vi "BCU诊断标定.vi"(8 "CAN端口":u16(ring), 9 "设备索引号":u16(ring), 10 "CAN卡类型":u32(ring)=21, 11 "Myindex":dbl=1.0) -> (3 "成功":bool)   [LabVIEW 2013] (continued)
                        n2401 = local write "风机继电器(从)"(w2943) -> ()
                        n2402 = One Button Dialog(message="继电器处理超时" ("消息"), button name ("OK")="是" ("按钮名称（“确定”）")) -> ()  [unwired: 1 out]
                      }
                      frame True {
                      }
                    }
                  }
                }
              }
            }
          }
          event "DO1": Value Change {
            n2403 = event-data() -> ("NewVal"=w2947:bool)  [unwired: 6 out]
            n2404 = stacked-sequence {
              tunnel: w2947 -> [_ w2960 _]
              frame #0 {
                w2950 = FALSE ("清BUFF")
                n2405 = local write "继电器超时处理"(FALSE ("继电器超时处理")) -> ()
                n2406 = local write "清BUFF"(w2950) -> ()
                n2407 = local write "正级继电器 9"(w2950) -> ()
                n2408 = local write "主从选择"(enum32{"主板", "从板"}."主板" ("主从选择")) -> ()
              }
              frame #1 {
                n2409 = case shown="真" w2960 {
                  selector: w2960 -> [w2975 w2995]
                  tunnel: [w2974 w2994] -> w2959
                  tunnel: [w2962 w2982] -> w2954
                  frame False {
                    w2970 = 256.0 ("y")
                    w2962 = u32 2 ("命令序号")
                    w2974 = u8 192 ("命令")
                    n2410 = local read "动作保持时间"() -> (w2971:dbl)
                    n2411 = Quotient & Remainder(x=w2971, y=w2970) -> (x-y*floor(x/y)=w2963:dbl, floor(x/y)=w2967:dbl)
                    n2412 = Quotient & Remainder(x=w2967, y=w2970) -> (x-y*floor(x/y)=w2964:dbl, floor(x/y)=w2968:dbl)
                    n2413 = Quotient & Remainder(x=w2968, y=w2970) -> (x-y*floor(x/y)=w2965:dbl, floor(x/y)=w2969:dbl)
                    n2414 = local read "设备索引号"() -> (w2979:u16)
                    n2415 = local read "CAN卡类型"() -> (w2980:u32)
                    n2416 = local read "CAN端口"() -> (w2978:u16)
                    n2417 = Boolean To (0,1)(Boolean=w2975) -> (0, 1=w2972:i16)
                    n2418 = Quotient & Remainder(x=w2969, y=w2970) -> (x-y*floor(x/y)=w2966:dbl)  [unwired: 1 out]
                    n2419 = Build Array(i16 1 ("元素"), w2972, w2966, w2965, w2964, w2963, 0.0 ("元素")) -> (w2976:dbl[])
                    n2420 = call "多帧发送机制(EV05).vi"("can卡类型"=w2980, "设备索引号"=w2979, "CAN端口"=w2978, "命令"=w2974, "板号"=u8 0, "命令序号"=w2962, "输入数据"=w2976) -> ()  [unwired: 2 in, 11 out]
                  }
                  frame True {
                    w2990 = 256.0 ("y")
                    w2982 = u32 2 ("命令序号")
                    w2994 = u8 192 ("命令")
                    n2421 = local read "动作保持时间"() -> (w2991:dbl)
                    n2422 = Quotient & Remainder(x=w2991, y=w2990) -> (x-y*floor(x/y)=w2983:dbl, floor(x/y)=w2987:dbl)
                    n2423 = Quotient & Remainder(x=w2987, y=w2990) -> (x-y*floor(x/y)=w2984:dbl, floor(x/y)=w2988:dbl)
                    n2424 = Quotient & Remainder(x=w2988, y=w2990) -> (x-y*floor(x/y)=w2985:dbl, floor(x/y)=w2989:dbl)
                    n2425 = local read "设备索引号"() -> (w2999:u16)
                    n2426 = local read "CAN卡类型"() -> (w3000:u32)
                    n2427 = local read "CAN端口"() -> (w2998:u16)
                    n2428 = Boolean To (0,1)(Boolean=w2995) -> (0, 1=w2992:i16)
                    n2429 = Quotient & Remainder(x=w2989, y=w2990) -> (x-y*floor(x/y)=w2986:dbl)  [unwired: 1 out]
                    n2430 = Build Array(i16 1 ("元素"), w2992, w2986, w2985, w2984, w2983, 0.0 ("元素")) -> (w2996:dbl[])
                    n2431 = call "多帧发送机制(EV05).vi"("can卡类型"=w3000, "设备索引号"=w2999, "CAN端口"=w2998, "命令"=w2994, "板号"=u8 0, "命令序号"=w2982, "输入数据"=w2996) -> ()  [unwired: 2 in, 11 out]
                  }
                }
                n2432 = local write "命令序号"(w2954) -> ()
                n2433 = local write "命令"(w2959) -> ()
                n2434 = local write "控制1"(TRUE ("控制1")) -> ()
                n2435 = local write "写?"(FALSE ("写?")) -> ()
                n2436 = local write "消除"(TRUE ("消除")) -> ()
                n2437 = global write "EV05全局变量1.vi" "流控帧 2"(TRUE ("流控帧 2")) -> ()
                n2438 = global write "EV05全局变量1.vi" "流控帧"(FALSE ("流控帧")) -> ()
              }
              frame #2 {
                n2439 = flat-sequence {
                  tunnel: [w3002] -> w3001
                  tunnel: w3001 -> [w3009]
                  frame #0 {
                    n2440 = while {
                      tunnel: [w3003] -> w3002
                      i -> [w3007]
                      stop <- w3004 stop-if-true
                      n2441 = local read "继电器超时处理"() -> (w3003:bool)
                      n2442 = Greater Or Equal?(x=w3007, y=20) -> (x >= y?=w3005:bool)
                      n2443 = Wait Until Next ms Multiple(millisecond multiple=u32 100 ("毫秒倍数")) -> ()  [unwired: 1 out]
                      n2444 = Or(x=w3003, y=w3005) -> (x .or. y?=w3004:bool)
                    }
                  }
                  frame #1 {
                    n2445 = case shown="假" w3009 {
                      frame False {
                        n2446 = local read "DO1"() -> (w3011:bool)
                        n2447 = Not(x=w3011) -> (.not. x?=w3010:bool)
                        n2448 = local write "DO1"(w3010) -> ()
                        n2449 = One Button Dialog(message="DO控制处理超时" ("消息"), button name ("OK")="是" ("按钮名称（“确定”）")) -> ()  [unwired: 1 out]
                      }
                      frame True {
                      }
                    }
                  }
                }
              }
            }
          }
          event "DO2": Value Change {
            n2450 = event-data() -> ("NewVal"=w3014:bool)  [unwired: 6 out]
            n2451 = stacked-sequence {
              tunnel: w3014 -> [_ w3027 _]
              frame #0 {
                w3017 = FALSE ("清BUFF")
                n2452 = local write "继电器超时处理"(FALSE ("继电器超时处理")) -> ()
                n2453 = local write "主从选择"(enum32{"主板", "从板"}."主板" ("主从选择")) -> ()
                n2454 = local write "清BUFF"(w3017) -> ()
                n2455 = local write "正级继电器 10"(w3017) -> ()
              }
              frame #1 {
                n2456 = case shown="真" w3027 {
                  selector: w3027 -> [w3042 w3062]
                  tunnel: [w3041 w3061] -> w3026
                  tunnel: [w3029 w3049] -> w3021
                  frame False {
                    w3037 = 256.0 ("y")
                    w3029 = u32 2 ("命令序号")
                    w3041 = u8 192 ("命令")
                    n2457 = local read "动作保持时间"() -> (w3038:dbl)
                    n2458 = Quotient & Remainder(x=w3038, y=w3037) -> (x-y*floor(x/y)=w3030:dbl, floor(x/y)=w3034:dbl)
                    n2459 = Quotient & Remainder(x=w3034, y=w3037) -> (x-y*floor(x/y)=w3031:dbl, floor(x/y)=w3035:dbl)
                    n2460 = Quotient & Remainder(x=w3035, y=w3037) -> (x-y*floor(x/y)=w3032:dbl, floor(x/y)=w3036:dbl)
                    n2461 = local read "设备索引号"() -> (w3046:u16)
                    n2462 = local read "CAN卡类型"() -> (w3047:u32)
                    n2463 = local read "CAN端口"() -> (w3045:u16)
                    n2464 = Boolean To (0,1)(Boolean=w3042) -> (0, 1=w3039:i16)
                    n2465 = Quotient & Remainder(x=w3036, y=w3037) -> (x-y*floor(x/y)=w3033:dbl)  [unwired: 1 out]
                    n2466 = Build Array(i16 2 ("元素"), w3039, w3033, w3032, w3031, w3030, 0.0 ("元素")) -> (w3043:dbl[])
                    n2467 = call "多帧发送机制(EV05).vi"("can卡类型"=w3047, "设备索引号"=w3046, "CAN端口"=w3045, "命令"=w3041, "板号"=u8 0, "命令序号"=w3029, "输入数据"=w3043) -> ()  [unwired: 2 in, 11 out]
                  }
                  frame True {
                    w3057 = 256.0 ("y")
                    w3049 = u32 2 ("命令序号")
                    w3061 = u8 192 ("命令")
                    n2468 = local read "动作保持时间"() -> (w3058:dbl)
                    n2469 = Quotient & Remainder(x=w3058, y=w3057) -> (x-y*floor(x/y)=w3050:dbl, floor(x/y)=w3054:dbl)
                    n2470 = Quotient & Remainder(x=w3054, y=w3057) -> (x-y*floor(x/y)=w3051:dbl, floor(x/y)=w3055:dbl)
                    n2471 = Quotient & Remainder(x=w3055, y=w3057) -> (x-y*floor(x/y)=w3052:dbl, floor(x/y)=w3056:dbl)
                    n2472 = local read "设备索引号"() -> (w3066:u16)
                    n2473 = local read "CAN卡类型"() -> (w3067:u32)
                    n2474 = local read "CAN端口"() -> (w3065:u16)
                    n2475 = Boolean To (0,1)(Boolean=w3062) -> (0, 1=w3059:i16)
                    n2476 = Quotient & Remainder(x=w3056, y=w3057) -> (x-y*floor(x/y)=w3053:dbl)  [unwired: 1 out]
                    n2477 = Build Array(i16 2 ("元素"), w3059, w3053, w3052, w3051, w3050, 0.0 ("元素")) -> (w3063:dbl[])
                    n2478 = call "多帧发送机制(EV05).vi"("can卡类型"=w3067, "设备索引号"=w3066, "CAN端口"=w3065, "命令"=w3061, "板号"=u8 0, "命令序号"=w3049, "输入数据"=w3063) -> ()  [unwired: 2 in, 11 out]
                  }
                }
                n2479 = local write "命令序号"(w3021) -> ()
                n2480 = local write "命令"(w3026) -> ()
                n2481 = local write "控制1"(TRUE ("控制1")) -> ()
                n2482 = local write "写?"(FALSE ("写?")) -> ()
                n2483 = local write "消除"(TRUE ("消除")) -> ()
                n2484 = global write "EV05全局变量1.vi" "流控帧 2"(TRUE ("流控帧 2")) -> ()
                n2485 = global write "EV05全局变量1.vi" "流控帧"(FALSE ("流控帧")) -> ()
              }
              frame #2 {
                n2486 = flat-sequence {
                  tunnel: [w3069] -> w3068
                  tunnel: w3068 -> [w3076]
                  frame #0 {
                    n2487 = while {
                      tunnel: [w3070] -> w3069
                      i -> [w3074]
                      stop <- w3071 stop-if-true
                      n2488 = local read "继电器超时处理"() -> (w3070:bool)
                      n2489 = Greater Or Equal?(x=w3074, y=20) -> (x >= y?=w3072:bool)
                      n2490 = Wait Until Next ms Multiple(millisecond multiple=u32 100 ("毫秒倍数")) -> ()  [unwired: 1 out]
                      n2491 = Or(x=w3070, y=w3072) -> (x .or. y?=w3071:bool)
                    }
                  }
                  frame #1 {
                    n2492 = case shown="假" w3076 {
                      frame False {
                        n2493 = local read "DO2"() -> (w3078:bool)
                        n2494 = Not(x=w3078) -> (.not. x?=w3077:bool)
                        n2495 = local write "DO2"(w3077) -> ()
                        n2496 = One Button Dialog(message="DO控制处理超时" ("消息"), button name ("OK")="是" ("按钮名称（“确定”）")) -> ()  [unwired: 1 out]
                      }
                      frame True {
                      }
                    }
                  }
                }
              }
            }
          }
          event "DO1 2": Value Change {
            n2497 = event-data() -> ("NewVal"=w3081:bool)  [unwired: 6 out]
            n2498 = stacked-sequence {
              tunnel: w3081 -> [_ w3095 _]
              frame #0 {
                w3084 = FALSE ("继电器超时处理")
                n2499 = local write "继电器超时处理"(w3084) -> ()
                n2500 = local write "正级继电器 11"(w3084) -> ()
                n2501 = local write "主从选择"(enum32{"主板", "从板"}."从板" ("主从选择")) -> ()
              }
              frame #1 {
                n2502 = case shown="假" w3095 {
                  selector: w3095 -> [w3110 w3130]
                  tunnel: [w3109 w3129] -> w3094
                  tunnel: [w3108 w3128] -> w3088
                  tunnel: [w3097 w3117] -> w3089
                  frame True {
                    w3105 = 256.0 ("y")
                    w3097 = u32 2 ("命令序号")
                    w3109 = u8 192 ("命令")
                    n2503 = local read "动作保持时间"() -> (w3106:dbl)
                    n2504 = Quotient & Remainder(x=w3106, y=w3105) -> (x-y*floor(x/y)=w3098:dbl, floor(x/y)=w3102:dbl)
                    n2505 = Quotient & Remainder(x=w3102, y=w3105) -> (x-y*floor(x/y)=w3099:dbl, floor(x/y)=w3103:dbl)
                    n2506 = Quotient & Remainder(x=w3103, y=w3105) -> (x-y*floor(x/y)=w3100:dbl, floor(x/y)=w3104:dbl)
                    n2507 = Quotient & Remainder(x=w3104, y=w3105) -> (x-y*floor(x/y)=w3101:dbl)  [unwired: 1 out]
                    n2508 = Boolean To (0,1)(Boolean=w3110) -> (0, 1=w3107:i16)
                    n2509 = local read "设备索引号"() -> (w3114:u16)
                    n2510 = local read "CAN卡类型"() -> (w3115:u32)
                    n2511 = local read "从板板号"() -> (w3108:u8)
                    n2512 = local read "CAN端口"() -> (w3113:u16)
                    n2513 = Build Array(i16 3 ("元素"), w3107, w3101, w3100, w3099, w3098, 0.0 ("元素")) -> (w3112:dbl[])
                    n2514 = call "多帧发送机制(EV05).vi"("can卡类型"=w3115, "设备索引号"=w3114, "CAN端口"=w3113, "命令"=w3109, "板号"=w3108, "命令序号"=w3097, "输入数据"=w3112) -> ()  [unwired: 2 in, 11 out]
                  }
                  frame False {
                    w3125 = 256.0 ("y")
                    w3117 = u32 2 ("命令序号")
                    w3129 = u8 192 ("命令")
                    n2515 = local read "动作保持时间"() -> (w3126:dbl)
                    n2516 = Quotient & Remainder(x=w3126, y=w3125) -> (x-y*floor(x/y)=w3118:dbl, floor(x/y)=w3122:dbl)
                    n2517 = Quotient & Remainder(x=w3122, y=w3125) -> (x-y*floor(x/y)=w3119:dbl, floor(x/y)=w3123:dbl)
                    n2518 = Quotient & Remainder(x=w3123, y=w3125) -> (x-y*floor(x/y)=w3120:dbl, floor(x/y)=w3124:dbl)
                    n2519 = Quotient & Remainder(x=w3124, y=w3125) -> (x-y*floor(x/y)=w3121:dbl)  [unwired: 1 out]
                    n2520 = Boolean To (0,1)(Boolean=w3130) -> (0, 1=w3127:i16)
                    n2521 = local read "设备索引号"() -> (w3134:u16)
                    n2522 = local read "CAN卡类型"() -> (w3135:u32)
                    n2523 = local read "从板板号"() -> (w3128:u8)
                    n2524 = local read "CAN端口"() -> (w3133:u16)
                    n2525 = Build Array(i16 1 ("元素"), w3127, w3121, w3120, w3119, w3118, 0.0 ("元素")) -> (w3132:dbl[])
                    n2526 = call "多帧发送机制(EV05).vi"("can卡类型"=w3135, "设备索引号"=w3134, "CAN端口"=w3133, "命令"=w3129, "板号"=w3128, "命令序号"=w3117, "输入数据"=w3132) -> ()  [unwired: 2 in, 11 out]
                  }
                }
                n2527 = local write "从板板号"(w3088) -> ()
                n2528 = local write "命令序号"(w3089) -> ()
                n2529 = local write "命令"(w3094) -> ()
                n2530 = local write "清BUFF"(FALSE ("清BUFF")) -> ()
                n2531 = local write "写?"(FALSE ("写?")) -> ()
                n2532 = local write "控制1"(TRUE ("控制1")) -> ()
                n2533 = global write "EV05全局变量1.vi" "流控帧"(FALSE ("流控帧")) -> ()
                n2534 = global write "EV05全局变量1.vi" "流控帧 2"(TRUE ("流控帧 2")) -> ()
                n2535 = local write "消除"(TRUE ("消除")) -> ()
              }
              frame #2 {
                n2536 = flat-sequence {
                  tunnel: [w3137] -> w3136
                  tunnel: w3136 -> [w3144]
                  frame #0 {
                    n2537 = while {
                      tunnel: [w3138] -> w3137
                      i -> [w3142]
                      stop <- w3139 stop-if-true
                      n2538 = local read "继电器超时处理"() -> (w3138:bool)
                      n2539 = Greater Or Equal?(x=w3142, y=20) -> (x >= y?=w3140:bool)
                      n2540 = Wait Until Next ms Multiple(millisecond multiple=u32 100 ("毫秒倍数")) -> ()  [unwired: 1 out]
                      n2541 = Or(x=w3138, y=w3140) -> (x .or. y?=w3139:bool)
                    }
                  }
                  frame #1 {
                    n2542 = case shown="假" w3144 {
                      frame False {
                        n2543 = local read "DO1 2"() -> (w3146:bool)
                        n2544 = Not(x=w3146) -> (.not. x?=w3145:bool)
                        n2545 = local write "DO1 2"(w3145) -> ()
                        n2546 = One Button Dialog(message="DO控制处理超时" ("消息"), button name ("OK")="是" ("按钮名称（“确定”）")) -> ()  [unwired: 1 out]
                      }
                      frame True {
                      }
                    }
                  }
                }
              }
            }
          }
          event "读取转换为写入": Value Change {
            n2547 = event-data() -> ("NewVal"=w3149:bool)  [unwired: 6 out]
            n2548 = case shown="真" w3149 {
              tunnel: w3153 -> [w3155 w3160]
              tunnel: [w3155 w3159] -> w3152
              tunnel: w3151 -> [w3154 w3158]
              tunnel: [w3154 w3157] -> w3150
              frame False {
              }
              frame True {
                n2549 = Enqueue Element(queue=w3160, element="读取转换为写入", error in (no error)=w3158) -> (queue out=w3159:refnum<queue>, error out=w3157:errorcluster)  [unwired: 2 out]
              }
            }
          }
          event "读取故障详细状态": Value Change {
            n2550 = event-data() -> ("NewVal"=w3165:bool)  [unwired: 5 out]
            n2551 = case shown="真" w3165 {
              tunnel: w3164 -> [w3167 w3180]
              tunnel: w3163 -> [w3166 w3179]
              tunnel: [w3167 w3178] -> w3162
              tunnel: [w3166 w3177] -> w3161
              frame False {
              }
              frame True {
                n2552 = disable-structure shown="启用" {
                  disable-tunnel: [w3189 TRUE ("发送成功")] -> w3176
                  frame Disabled {
                    n2553 = local read "主从选择"() -> (w3181:enum32{"主板", "从板"})
                    n2554 = case shown="\"主板\", 默认" w3181 {
                      tunnel: [0.0 ("FUNC") w3191] -> w3186
                      frame "主板", Default {
                      }
                      frame "从板" {
                        n2555 = local read "从板号"() -> (w3191:u8)
                      }
                    }
                    n2556 = local read "设备索引号"() -> (w3183:u16)
                    n2557 = local read "CAN卡类型"() -> (w3184:u32)
                    n2558 = local read "CAN端口"() -> (w3182:u16)
                    n2559 = call "标定授权发送.vi"("CAN卡类型"=w3184, "解锁类型"=enum16{"读取", "写", "下载"}."写", "设备索引号"=w3183, "CAN端口"=w3182, "是否连接"=TRUE, "板选择"=0, "FUNC"=w3186) -> ("发送成功"=w3189:bool)  [unwired: 8 out]
                  }
                  frame Enabled {
                  }
                }
                n2560 = case shown="真" w3176 {
                  tunnel: w3180 -> [w3194 w3199]
                  tunnel: w3179 -> [w3193 w3198]
                  tunnel: [w3194 w3196] -> w3178
                  tunnel: [w3193 w3195] -> w3177
                  frame False {
                  }
                  frame True {
                    n2561 = Enqueue Element(queue=w3199, element="读取故障状态" ("元素"), error in (no error)=w3198) -> (queue out=w3196:refnum<queue>, error out=w3195:errorcluster)  [unwired: 2 out]
                  }
                }
                n2562 = local write "电池故障"(string[][] []) -> ()
                n2563 = global write "EV05全局变量1.vi" "流控帧 2"(TRUE ("流控帧")) -> ()
                n2564 = local write "写?"(FALSE ("写?")) -> ()
                n2565 = local write "控制1"(TRUE ("控制1")) -> ()
                n2566 = local write "消除"(TRUE ("消除")) -> ()
                n2567 = local write "清BUFF"(FALSE ("清BUFF")) -> ()
                n2568 = global write "EV05全局变量1.vi" "流控帧"(FALSE ("流控帧")) -> ()
                n2569 = call <vilib>:"Set Busy.vi"("disable click? (T)"=FALSE) -> ()  [unwired: 3 in, 8 out]
              }
            }
          }
          event "项目软本读取": Value Change {
            n2570 = event-data() -> ("NewVal"=w3204:bool)  [unwired: 5 out]
            n2571 = case shown="真" w3204 {
              tunnel: w3203 -> [w3206 w3213]
              tunnel: w3202 -> [w3205 w3212]
              tunnel: [w3206 w3211] -> w3201
              tunnel: [w3205 w3210] -> w3200
              frame False {
              }
              frame True {
                n2572 = global read "EV05全局变量1.vi" "授权功能"() -> (w3208:bool)
                n2573 = case shown="假" w3208 {
                  tunnel: [TRUE ("发送成功") w3232] -> w3209
                  frame False {
                  }
                  frame True {
                    n2574 = local read "设备索引号"() -> (w3227:u16)
                    n2575 = local read "CAN卡类型"() -> (w3228:u32)
                    n2576 = local read "CAN端口"() -> (w3226:u16)
                    n2577 = call "标定授权发送.vi"("CAN卡类型"=w3228, "解锁类型"=enum16{"读取", "写", "下载"}."读取", "设备索引号"=w3227, "CAN端口"=w3226, "是否连接"=TRUE, "板选择"=0, "FUNC"=u32 0) -> ("发送成功"=w3232:bool)  [unwired: 8 out]
                  }
                }
                n2578 = stacked-sequence {
                  tunnel: [w3216] -> w3207
                  frame #0 {
                    w3216 = FALSE ("disable click? (T)")
                    w3219 = FALSE ("写?")
                    n2579 = local write "写?"(w3219) -> ()
                    n2580 = global write "EV05全局变量1.vi" "写入超时"(w3219) -> ()
                    n2581 = local write "项目软件版本号"(" " ("项目软件版本号")) -> ()
                    n2582 = global write "EV05全局变量1.vi" "流控帧"(FALSE ("流控帧")) -> ()
                    n2583 = local write "主从选择"(enum32{"主板", "从板"}."主板" ("主从选择")) -> ()
                    n2584 = call <vilib>:"Set Busy.vi"("disable click? (T)"=w3216) -> ()  [unwired: 3 in, 8 out]
                    n2585 = local write "清BUFF"(FALSE ("清BUFF")) -> ()
                    n2586 = property on="保存版本信息" class="Bool (严格)"("Visible"=TRUE ("可见")) -> ()  [unwired: 2 in, 2 out]
                    n2587 = global write "EV05全局变量1.vi" "流控帧 2"(TRUE ("流控帧 2")) -> ()
                    n2588 = local write "控制1"(TRUE ("控制1")) -> ()
                    n2589 = local write "消除"(TRUE ("消除")) -> ()
                  }
                }
                n2590 = case shown="真" w3209 {
                  tunnel: w3213 -> [w3234 w3239]
                  tunnel: w3212 -> [w3233 w3238]
                  tunnel: [w3234 w3236] -> w3211
                  tunnel: [w3233 w3235] -> w3210
                  tunnel: w3207 -> [_ _]
                  frame False {
                  }
                  frame True {
                    n2591 = Enqueue Element(queue=w3239, element="项目软件版本读取" ("元素"), error in (no error)=w3238) -> (queue out=w3236:refnum<queue>, error out=w3235:errorcluster)  [unwired: 2 out]
                  }
                }
              }
            }
          }
          event "读硬件版本号": Value Change {
            n2592 = event-data() -> ("NewVal"=w3244:bool)  [unwired: 5 out]
            n2593 = case shown="真" w3244 {
              tunnel: w3243 -> [w3246 w3253]
              tunnel: w3242 -> [w3245 w3252]
              tunnel: [w3246 w3251] -> w3241
              tunnel: [w3245 w3250] -> w3240
              frame False {
              }
              frame True {
                n2594 = global read "EV05全局变量1.vi" "授权功能"() -> (w3248:bool)
                n2595 = case shown="假" w3248 {
                  tunnel: [TRUE ("发送成功") w3272] -> w3249
                  frame False {
                  }
                  frame True {
                    n2596 = local read "设备索引号"() -> (w3267:u16)
                    n2597 = local read "CAN卡类型"() -> (w3268:u32)
                    n2598 = local read "CAN端口"() -> (w3266:u16)
                    n2599 = call "标定授权发送.vi"("CAN卡类型"=w3268, "解锁类型"=enum16{"读取", "写", "下载"}."读取", "设备索引号"=w3267, "CAN端口"=w3266, "是否连接"=TRUE, "板选择"=0, "FUNC"=u32 0) -> ("发送成功"=w3272:bool)  [unwired: 8 out]
                  }
                }
                n2600 = stacked-sequence {
                  tunnel: [w3256] -> w3247
                  frame #0 {
                    w3256 = TRUE ("控制1")
                    w3260 = FALSE ("写?")
                    n2601 = local write "写?"(w3260) -> ()
                    n2602 = global write "EV05全局变量1.vi" "写入超时"(w3260) -> ()
                    n2603 = call <vilib>:"Set Busy.vi"("disable click? (T)"=FALSE) -> ()  [unwired: 3 in, 8 out]
                    n2604 = local write "硬件版本号"("" ("硬件版本号")) -> ()
                    n2605 = property on="保存版本信息" class="Bool (严格)"("Visible"=TRUE ("可见")) -> ()  [unwired: 2 in, 2 out]
                    n2606 = local write "主从选择"(enum32{"主板", "从板"}."主板" ("主从选择")) -> ()
                    n2607 = local write "控制1"(w3256) -> ()
                    n2608 = local write "清BUFF"(FALSE ("清BUFF")) -> ()
                    n2609 = global write "EV05全局变量1.vi" "流控帧 2"(TRUE ("流控帧 2")) -> ()
                    n2610 = local write "消除"(TRUE ("消除")) -> ()
                    n2611 = global write "EV05全局变量1.vi" "流控帧"(FALSE ("流控帧")) -> ()
                  }
                }
                n2612 = case shown="真" w3249 {
                  tunnel: w3253 -> [w3274 w3279]
                  tunnel: w3252 -> [w3273 w3278]
                  tunnel: [w3274 w3276] -> w3251
                  tunnel: [w3273 w3275] -> w3250
                  tunnel: w3247 -> [_ _]
                  frame False {
                  }
                  frame True {
                    n2613 = Enqueue Element(queue=w3279, element="硬件版本读取" ("元素"), error in (no error)=w3278) -> (queue out=w3276:refnum<queue>, error out=w3275:errorcluster)  [unwired: 2 out]
                  }
                }
              }
            }
          }
          event "平台软件版本读取": Value Change {
            n2614 = event-data() -> ("NewVal"=w3284:bool)  [unwired: 5 out]
            n2615 = case shown="真" w3284 {
              tunnel: w3283 -> [w3286 w3293]
              tunnel: w3282 -> [w3285 w3292]
              tunnel: [w3286 w3291] -> w3281
              tunnel: [w3285 w3290] -> w3280
              frame False {
              }
              frame True {
                n2616 = global read "EV05全局变量1.vi" "授权功能"() -> (w3288:bool)
                n2617 = case shown="假" w3288 {
                  tunnel: [TRUE ("发送成功") w3312] -> w3289
                  frame False {
                  }
                  frame True {
                    n2618 = local read "设备索引号"() -> (w3307:u16)
                    n2619 = local read "CAN卡类型"() -> (w3308:u32)
                    n2620 = local read "CAN端口"() -> (w3306:u16)
                    n2621 = call "标定授权发送.vi"("CAN卡类型"=w3308, "解锁类型"=enum16{"读取", "写", "下载"}."读取", "设备索引号"=w3307, "CAN端口"=w3306, "是否连接"=TRUE, "板选择"=0, "FUNC"=u32 0) -> ("发送成功"=w3312:bool)  [unwired: 8 out]
                  }
                }
                n2622 = stacked-sequence {
                  tunnel: [w3296] -> w3287
                  frame #0 {
                    w3296 = TRUE ("控制1")
                    w3300 = FALSE ("写?")
                    n2623 = call <vilib>:"Set Busy.vi"("disable click? (T)"=FALSE) -> ()  [unwired: 3 in, 8 out]
                    n2624 = local write "写?"(w3300) -> ()
                    n2625 = global write "EV05全局变量1.vi" "写入超时"(w3300) -> ()
                    n2626 = local write "平台软件版本号"(" " ("平台软件版本号")) -> ()
                    n2627 = local write "控制1"(w3296) -> ()
                    n2628 = local write "消除"(TRUE ("消除")) -> ()
                    n2629 = property on="保存版本信息" class="Bool (严格)"("Visible"=TRUE ("可见")) -> ()  [unwired: 2 in, 2 out]
                    n2630 = global write "EV05全局变量1.vi" "流控帧 2"(TRUE ("流控帧 2")) -> ()
                    n2631 = local write "主从选择"(enum32{"主板", "从板"}."主板" ("主从选择")) -> ()
                    n2632 = local write "清BUFF"(FALSE ("清BUFF")) -> ()
                    n2633 = global write "EV05全局变量1.vi" "流控帧"(FALSE ("流控帧")) -> ()
                  }
                }
                n2634 = case shown="真" w3289 {
                  tunnel: w3293 -> [w3314 w3319]
                  tunnel: w3292 -> [w3313 w3318]
                  tunnel: [w3314 w3316] -> w3291
                  tunnel: [w3313 w3315] -> w3290
                  tunnel: w3287 -> [_ _]
                  frame False {
                  }
                  frame True {
                    n2635 = Enqueue Element(queue=w3319, element="平台软件版本读取" ("元素"), error in (no error)=w3318) -> (queue out=w3316:refnum<queue>, error out=w3315:errorcluster)  [unwired: 2 out]
                  }
                }
              }
            }
          }
          event "模块版本读取": Value Change {
            n2636 = event-data() -> ("NewVal"=w3324:bool)  [unwired: 5 out]
            n2637 = case shown="真" w3324 {
              tunnel: w3323 -> [w3326 w3333]
              tunnel: w3322 -> [w3325 w3332]
              tunnel: [w3326 w3331] -> w3321
              tunnel: [w3325 w3330] -> w3320
              frame False {
              }
              frame True {
                n2638 = global read "EV05全局变量1.vi" "授权功能"() -> (w3328:bool)
                n2639 = case shown="假" w3328 {
                  tunnel: [TRUE ("发送成功") w3351] -> w3329
                  frame False {
                  }
                  frame True {
                    n2640 = local read "设备索引号"() -> (w3346:u16)
                    n2641 = local read "CAN卡类型"() -> (w3347:u32)
                    n2642 = local read "CAN端口"() -> (w3345:u16)
                    n2643 = call "标定授权发送.vi"("CAN卡类型"=w3347, "解锁类型"=enum16{"读取", "写", "下载"}."读取", "设备索引号"=w3346, "CAN端口"=w3345, "是否连接"=TRUE, "板选择"=0, "FUNC"=u32 0) -> ("发送成功"=w3351:bool)  [unwired: 8 out]
                  }
                }
                n2644 = stacked-sequence {
                  tunnel: [w3336] -> w3327
                  frame #0 {
                    w3336 = TRUE ("控制1")
                    w3339 = FALSE ("写?")
                    n2645 = call <vilib>:"Set Busy.vi"("disable click? (T)"=FALSE) -> ()  [unwired: 3 in, 8 out]
                    n2646 = local write "写?"(w3339) -> ()
                    n2647 = global write "EV05全局变量1.vi" "写入超时"(w3339) -> ()
                    n2648 = local write "主从选择"(enum32{"主板", "从板"}."主板" ("主从选择")) -> ()
                    n2649 = local write "清BUFF"(FALSE ("清BUFF")) -> ()
                    n2650 = property on="保存版本信息" class="Bool (严格)"("Visible"=TRUE ("可见")) -> ()  [unwired: 2 in, 2 out]
                    n2651 = global write "EV05全局变量1.vi" "流控帧 2"(TRUE ("流控帧 2")) -> ()
                    n2652 = local write "控制1"(w3336) -> ()
                    n2653 = local write "消除"(TRUE ("消除")) -> ()
                    n2654 = global write "EV05全局变量1.vi" "流控帧"(FALSE ("流控帧")) -> ()
                  }
                }
                n2655 = case shown="真" w3329 {
                  tunnel: w3333 -> [w3353 w3358]
                  tunnel: w3332 -> [w3352 w3357]
                  tunnel: [w3353 w3355] -> w3331
                  tunnel: [w3352 w3354] -> w3330
                  tunnel: w3327 -> [_ _]
                  frame False {
                  }
                  frame True {
                    n2656 = Enqueue Element(queue=w3358, element="模块软件版本读取" ("元素"), error in (no error)=w3357) -> (queue out=w3355:refnum<queue>, error out=w3354:errorcluster)  [unwired: 2 out]
                  }
                }
              }
            }
          }
          event "保存版本信息": Value Change {
            n2657 = event-data() -> ("NewVal"=w3359:bool)  [unwired: 6 out]
            n2658 = case shown="真" w3359 {
              frame False {
              }
              frame True {
                n2659 = stacked-sequence {
                  seq-local: [w3363 _] -> [_ w3365]
                  seq-local: [w3362 _] -> [_ w3364]
                  frame #0 {
                    n2660 = call "请输入从板个数"() -> ("从板个数"=w3363:dbl, "确定"=w3362:bool)  [unwired: 17 in, 1 out]
                  }
                  frame #1 {
                    n2661 = case shown="真" w3364 {
                      tunnel: w3365 -> [_ w3368]
                      frame False {
                      }
                      frame True {
                        n2662 = call <vilib>:"Application Directory.vi"() -> ("Application Directory"=w3380:path)
                        n2663 = Build Path(base path=w3380, name or relative path="SaveData" ("名称或相对路径")) -> (appended path=w3378:path)
                        n2664 = local read "模块版本名称"() -> (w3373:string[][])
                        n2665 = local read "项目软件版本"() -> (w3370:string[])
                        n2666 = local read "模块版本值"() -> (w3372:string[][])
                        n2667 = local read "平台软件版本"() -> (w3369:string[])
                        n2668 = local read "模块个数"() -> (w3366:u8[])
                        n2669 = local read "硬件版本"() -> (w3371:string[])
                        n2670 = call "文件对话框3"("start path"=w3378, "prompt"="选择要保存数据的位置", "default name"="BMS版本信息.txt") -> ("selected path"=w3374:path, "cancelled"=w3375:bool)  [unwired: 9 in, 2 out]
                        n2671 = Increment(x=w3368) -> (x+1=w3367:dbl)
                        n2672 = for {
                          N: w3367 -> [_]
                          tunnel: w3375 -> [w3396]
                          tunnel: w3374 -> [w3395]
                          tunnel: w3373 -> [w3385] mode=indexing
                          tunnel: w3372 -> [w3383] mode=indexing
                          tunnel: w3371 -> [w3390] mode=indexing
                          tunnel: w3370 -> [w3389] mode=indexing
                          tunnel: w3369 -> [w3388] mode=indexing
                          tunnel: w3366 -> [w3381] mode=indexing
                          i -> [w3387]
                          w3393 = ""
                          w3400 = 0 ("索引")
                          n2673 = case shown="0, 默认" w3387 {
                            selector: w3387 -> [_ w3414]
                            tunnel: ["主板版本信息" w3415] -> w3405
                            tunnel: [FALSE TRUE] -> w3391
                            frame 0, Default {
                            }
                            frame 1.. {
                              n2674 = Number To Decimal String(number=w3414) -> (decimal integer string=w3413:string)  [unwired: 1 in]
                              n2675 = Concatenate Strings("从板", w3413, "版本信息") -> (w3415:string)
                            }
                          }
                          n2676 = Increment(x=w3381) -> (x+1=w3382:u8)
                          n2677 = Array Subset(array=w3385, length=w3382) -> (w3386:string[])  [unwired: 1 in]
                          n2678 = Array Subset(array=w3383, length=w3382) -> (w3384:string[])  [unwired: 1 in]
                          n2679 = Build Array(w3393, w3388, w3389, w3390, w3393) -> (w3399:string[])
                          n2680 = Build Array(w3405, "平台软件版本号", "项目软件版本号", "硬件版本号", "模块版本号") -> (w3401:string[])
                          n2681 = Insert Into Array(array=w3386, index=w3400, new element=w3401) -> (w3398:string[])
                          n2682 = Insert Into Array(array=w3384, index=w3400, new element=w3399) -> (w3397:string[])
                          n2683 = Build Array(w3398, w3397) -> (w3394:string[][])
                          n2684 = case shown="假" w3396 {
                            tunnel: w3395 -> [w3409 _]
                            tunnel: w3394 -> [w3408 _]
                            tunnel: w3391 -> [w3406 _]
                            frame False {
                              n2685 = call-poly <vilib>:"Write To Spreadsheet File.vi"("transpose? (no:F)"=TRUE, "append to file? (new file:F)"=w3406, "2D data"=w3408, "file path (dialog if empty)"=w3409) -> ()  [unwired: 4 in, 1 out]
                            }
                            frame True {
                            }
                          }
                        }
                      }
                    }
                  }
                }
              }
            }
          }
          event "单个写入": Value Change {
            n2686 = event-data() -> ("NewVal"=w3422:bool)  [unwired: 5 out]
            n2687 = case shown="真" w3422 {
              tunnel: w3421 -> [w3424 w3431]
              tunnel: w3420 -> [w3423 w3430]
              tunnel: [w3424 w3429] -> w3419
              tunnel: [w3423 w3428] -> w3418
              frame False {
              }
              frame True {
                w3426 = FALSE ("流控帧")
                w3425 = TRUE ("流控帧 2")
                n2688 = disable-structure shown="启用" {
                  disable-tunnel: [w3440 TRUE ("发送成功")] -> w3427
                  frame Disabled {
                    n2689 = local read "主从选择"() -> (w3432:enum32{"主板", "从板"})
                    n2690 = case shown="\"主板\", 默认" w3432 {
                      tunnel: [0.0 ("FUNC") w3442] -> w3437
                      frame "主板", Default {
                      }
                      frame "从板" {
                        n2691 = local read "从板号"() -> (w3442:u8)
                      }
                    }
                    n2692 = local read "设备索引号"() -> (w3434:u16)
                    n2693 = local read "CAN卡类型"() -> (w3435:u32)
                    n2694 = local read "CAN端口"() -> (w3433:u16)
                    n2695 = call "标定授权发送.vi"("CAN卡类型"=w3435, "解锁类型"=enum16{"读取", "写", "下载"}."写", "设备索引号"=w3434, "CAN端口"=w3433, "是否连接"=TRUE, "板选择"=0, "FUNC"=w3437) -> ("发送成功"=w3440:bool)  [unwired: 8 out]
                  }
                  frame Enabled {
                  }
                }
                n2696 = case shown="真" w3427 {
                  tunnel: w3431 -> [w3445 w3449]
                  tunnel: w3430 -> [w3444 w3448]
                  tunnel: [w3445 w3451] -> w3429
                  tunnel: [w3444 w3450] -> w3428
                  frame False {
                  }
                  frame True {
                    n2697 = Flush Queue(queue=w3449, error in (no error)=w3448) -> (queue out=w3447:refnum<queue>, error out=w3446:errorcluster)  [unwired: 1 out]
                    n2698 = Enqueue Element(queue=w3447, element="单个写入" ("元素"), error in (no error)=w3446) -> (queue out=w3451:refnum<queue>, error out=w3450:errorcluster)  [unwired: 2 out]
                  }
                }
                n2699 = global write "EV05全局变量1.vi" "读取超时"(w3426) -> ()
                n2700 = global write "EV05全局变量1.vi" "流控帧"(w3426) -> ()
                n2701 = local write "消除"(w3425) -> ()
                n2702 = local write "控制1"(w3425) -> ()
                n2703 = global write "EV05全局变量1.vi" "流控帧 2"(w3425) -> ()
                n2704 = local write "写?"(w3425) -> ()
              }
            }
          }
          event "全部写入": Value Change {
            n2705 = event-data() -> ("NewVal"=w3457:bool)  [unwired: 5 out]
            n2706 = case shown="真" w3457 {
              tunnel: w3456 -> [w3459 w3467]
              tunnel: w3455 -> [w3458 w3466]
              tunnel: [w3459 w3465] -> w3454
              tunnel: [w3458 w3464] -> w3453
              frame False {
              }
              frame True {
                w3461 = FALSE ("流控帧")
                w3460 = TRUE ("流控帧 2")
                n2707 = global read "EV05全局变量1.vi" "授权功能"() -> (w3462:bool)
                n2708 = case shown="真" w3462 {
                  tunnel: [TRUE ("发送成功") w3477] -> w3463
                  frame False {
                  }
                  frame True {
                    n2709 = local read "主从选择"() -> (w3469:enum32{"主板", "从板"})
                    n2710 = case shown="\"从板\"" w3469 {
                      tunnel: [0.0 ("FUNC") w3479] -> w3470
                      frame "主板", Default {
                      }
                      frame "从板" {
                        n2711 = local read "从板号"() -> (w3479:u8)
                      }
                    }
                    n2712 = local read "设备索引号"() -> (w3472:u16)
                    n2713 = local read "CAN卡类型"() -> (w3473:u32)
                    n2714 = local read "CAN端口"() -> (w3471:u16)
                    n2715 = call "标定授权发送.vi"("CAN卡类型"=w3473, "解锁类型"=enum16{"读取", "写", "下载"}."写", "设备索引号"=w3472, "CAN端口"=w3471, "是否连接"=TRUE, "板选择"=0, "FUNC"=w3470) -> ("发送成功"=w3477:bool)  [unwired: 8 out]
                  }
                }
                n2716 = case shown="真" w3463 {
                  tunnel: w3467 -> [w3481 w3485]
                  tunnel: w3466 -> [w3480 w3484]
                  tunnel: [w3481 w3487] -> w3465
                  tunnel: [w3480 w3486] -> w3464
                  frame False {
                  }
                  frame True {
                    n2717 = Flush Queue(queue=w3485, error in (no error)=w3484) -> (queue out=w3483:refnum<queue>, error out=w3482:errorcluster)  [unwired: 1 out]
                    n2718 = Enqueue Element(queue=w3483, element="全部写入" ("元素"), error in (no error)=w3482) -> (queue out=w3487:refnum<queue>, error out=w3486:errorcluster)  [unwired: 1 in, 1 out]
                  }
                }
                n2719 = global write "EV05全局变量1.vi" "读取超时"(w3461) -> ()
                n2720 = global write "EV05全局变量1.vi" "流控帧"(w3461) -> ()
                n2721 = local write "消除"(w3460) -> ()
                n2722 = local write "控制1"(w3460) -> ()
                n2723 = global write "EV05全局变量1.vi" "流控帧 2"(w3460) -> ()
                n2724 = local write "写?"(w3460) -> ()
              }
            }
          }
          event "单个读取": Value Change {
            n2725 = event-data() -> ("NewVal"=w3493:bool)  [unwired: 5 out]
            n2726 = case shown="真" w3493 {
              tunnel: w3492 -> [w3495 w3503]
              tunnel: w3491 -> [w3494 w3502]
              tunnel: [w3495 w3501] -> w3490
              tunnel: [w3494 w3500] -> w3489
              frame False {
              }
              frame True {
                w3496 = FALSE ("流控帧")
                w3497 = TRUE ("流控帧 2")
                n2727 = global read "EV05全局变量1.vi" "授权功能"() -> (w3498:bool)
                n2728 = case shown="假" w3498 {
                  tunnel: [TRUE ("发送成功") w3512] -> w3499
                  frame False {
                  }
                  frame True {
                    n2729 = local read "设备索引号"() -> (w3506:u16)
                    n2730 = local read "CAN卡类型"() -> (w3507:u32)
                    n2731 = local read "CAN端口"() -> (w3505:u16)
                    n2732 = call "标定授权发送.vi"("CAN卡类型"=w3507, "解锁类型"=enum16{"读取", "写", "下载"}."读取", "设备索引号"=w3506, "CAN端口"=w3505, "是否连接"=TRUE, "板选择"=0, "FUNC"=u32 1) -> ("发送成功"=w3512:bool)  [unwired: 8 out]
                  }
                }
                n2733 = case shown="真" w3499 {
                  tunnel: w3503 -> [w3514 w3518]
                  tunnel: w3502 -> [w3513 w3516]
                  tunnel: [w3514 w3520] -> w3501
                  tunnel: [w3513 w3519] -> w3500
                  frame False {
                  }
                  frame True {
                    n2734 = Flush Queue(queue=w3518, error in (no error)=w3516) -> (queue out=w3517:refnum<queue>, error out=w3515:errorcluster)  [unwired: 1 out]
                    n2735 = Enqueue Element(queue=w3517, element="单个读取" ("元素"), error in (no error)=w3515) -> (queue out=w3520:refnum<queue>, error out=w3519:errorcluster)  [unwired: 2 out]
                  }
                }
                n2736 = global write "EV05全局变量1.vi" "写入超时"(w3496) -> ()
                n2737 = global write "EV05全局变量1.vi" "流控帧"(w3496) -> ()
                n2738 = local write "写?"(w3496) -> ()
                n2739 = local write "消除"(w3497) -> ()
                n2740 = local write "控制1"(w3497) -> ()
                n2741 = global write "EV05全局变量1.vi" "流控帧 2"(w3497) -> ()
              }
            }
          }
          event "全部读取": Value Change {
            n2742 = event-data() -> ("NewVal"=w3526:bool)  [unwired: 5 out]
            n2743 = case shown="真" w3526 {
              tunnel: w3525 -> [w3528 w3532]
              tunnel: w3524 -> [w3527 w3531]
              tunnel: [w3528 w3530] -> w3523
              tunnel: [w3527 w3529] -> w3522
              frame False {
              }
              frame True {
                n2744 = stacked-sequence {
                  seq-local: [w3537 _] -> [_ _]
                  seq-local: [w3536 _] -> [_ _]
                  tunnel: w3532 -> [w3539 w3569]
                  tunnel: w3531 -> [w3538 w3568]
                  tunnel: [_ w3573] -> w3530
                  tunnel: [_ w3572] -> w3529
                  frame #0 {
                    w3533 = FALSE ("布尔")
                    n2745 = local read "路径"() -> (w3535:path)
                    n2746 = Empty String/Path?(string/path=w3535) -> (empty?=w3534:bool)
                    n2747 = case shown="假" w3534 {
                      tunnel: w3539 -> [w3547 w3565]
                      tunnel: w3538 -> [w3546 w3564]
                      tunnel: [w3543 w3564] -> w3537
                      tunnel: [w3542 w3565] -> w3536
                      frame False {
                        n2748 = global read "EV05全局变量1.vi" "授权功能"() -> (w3544:bool)
                        n2749 = case shown="真" w3544 {
                          tunnel: [TRUE ("发送成功") w3556] -> w3545
                          frame False {
                          }
                          frame True {
                            n2750 = local read "设备索引号"() -> (w3550:u16)
                            n2751 = local read "CAN卡类型"() -> (w3551:u32)
                            n2752 = local read "CAN端口"() -> (w3549:u16)
                            n2753 = call "标定授权发送.vi"("CAN卡类型"=w3551, "解锁类型"=enum16{"读取", "写", "下载"}."读取", "设备索引号"=w3550, "CAN端口"=w3549, "是否连接"=TRUE, "板选择"=0, "FUNC"=u32 1) -> ("发送成功"=w3556:bool)  [unwired: 8 out]
                          }
                        }
                        n2754 = case shown="真" w3545 {
                          tunnel: w3547 -> [w3558 w3563]
                          tunnel: w3546 -> [w3557 w3562]
                          tunnel: [w3558 w3560] -> w3542
                          tunnel: [w3557 w3559] -> w3543
                          frame False {
                          }
                          frame True {
                            n2755 = Enqueue Element(queue=w3563, element="读配置文件" ("元素"), error in (no error)=w3562) -> (queue out=w3560:refnum<queue>, error out=w3559:errorcluster)  [unwired: 2 out]
                          }
                        }
                        n2756 = local write "布尔"(FALSE ("布尔")) -> ()
                        n2757 = Wait Until Next ms Multiple(millisecond multiple=u32 200 ("毫秒倍数")) -> ()  [unwired: 1 out]
                      }
                      frame True {
                      }
                    }
                    n2758 = local write "1 6"(w3533) -> ()
                    n2759 = local write "1 7"(w3533) -> ()
                    n2760 = local write "1 8"(w3533) -> ()
                    n2761 = local write "1 9"(w3533) -> ()
                    n2762 = local write "1 10"(w3533) -> ()
                    n2763 = local write "1 12"(w3533) -> ()
                  }
                  frame #1 {
                    w3566 = FALSE ("流控帧")
                    w3567 = TRUE ("流控帧 2")
                    n2764 = global read "EV05全局变量1.vi" "授权功能"() -> (w3570:bool)
                    n2765 = case shown="假" w3570 {
                      tunnel: [TRUE ("发送成功") w3582] -> w3571
                      frame False {
                      }
                      frame True {
                        n2766 = local read "设备索引号"() -> (w3576:u16)
                        n2767 = local read "CAN卡类型"() -> (w3577:u32)
                        n2768 = local read "CAN端口"() -> (w3575:u16)
                        n2769 = call "标定授权发送.vi"("CAN卡类型"=w3577, "解锁类型"=enum16{"读取", "写", "下载"}."读取", "设备索引号"=w3576, "CAN端口"=w3575, "是否连接"=TRUE, "板选择"=0, "FUNC"=u32 1) -> ("发送成功"=w3582:bool)  [unwired: 8 out]
                      }
                    }
                    n2770 = case shown="真" w3571 {
                      tunnel: w3569 -> [w3584 w3585]
                      tunnel: w3568 -> [w3583 w3588]
                      tunnel: [w3584 w3590] -> w3573
                      tunnel: [w3583 w3589] -> w3572
                      frame False {
                      }
                      frame True {
                        n2771 = Flush Queue(queue=w3585, error in (no error)=w3588) -> (queue out=w3586:refnum<queue>, error out=w3587:errorcluster)  [unwired: 1 out]
                        n2772 = Enqueue Element(queue=w3586, element="全部读取" ("元素"), error in (no error)=w3587) -> (queue out=w3590:refnum<queue>, error out=w3589:errorcluster)  [unwired: 2 out]
                      }
                    }
                    n2773 = global write "EV05全局变量1.vi" "写入超时"(w3566) -> ()
                    n2774 = global write "EV05全局变量1.vi" "流控帧"(w3566) -> ()
                    n2775 = local write "写?"(w3566) -> ()
                    n2776 = local write "消除"(w3567) -> ()
                    n2777 = local write "控制1"(w3567) -> ()
                    n2778 = global write "EV05全局变量1.vi" "流控帧 2"(w3567) -> ()
                  }
                }
              }
            }
          }
          event "开启均衡": Value Change {
            n2779 = event-data() -> ("NewVal"=w3596:bool)  [unwired: 5 out]
            n2780 = case shown="真" w3596 {
              tunnel: w3595 -> [w3598 w3605]
              tunnel: w3594 -> [w3597 w3604]
              tunnel: [w3598 w3603] -> w3593
              tunnel: [w3597 w3602] -> w3592
              frame False {
              }
              frame True {
                n2781 = global read "EV05全局变量1.vi" "授权功能"() -> (w3600:bool)
                n2782 = case shown="假" w3600 {
                  tunnel: [TRUE ("发送成功") w3615] -> w3601
                  frame False {
                  }
                  frame True {
                    n2783 = local read "主从选择"() -> (w3607:enum32{"主板", "从板"})
                    n2784 = case shown="\"从板\"" w3607 {
                      tunnel: [0.0 ("FUNC") w3617] -> w3608
                      frame "主板", Default {
                      }
                      frame "从板" {
                        n2785 = local read "从板号"() -> (w3617:u8)
                      }
                    }
                    n2786 = local read "设备索引号"() -> (w3610:u16)
                    n2787 = local read "CAN卡类型"() -> (w3611:u32)
                    n2788 = local read "CAN端口"() -> (w3609:u16)
                    n2789 = call "标定授权发送.vi"("CAN卡类型"=w3611, "解锁类型"=enum16{"读取", "写", "下载"}."写", "设备索引号"=w3610, "CAN端口"=w3609, "是否连接"=TRUE, "板选择"=0, "FUNC"=w3608) -> ("发送成功"=w3615:bool)  [unwired: 8 out]
                  }
                }
                n2790 = case shown="真" w3601 {
                  tunnel: w3605 -> [w3619 w3624]
                  tunnel: w3604 -> [w3618 w3623]
                  tunnel: [w3619 w3621] -> w3603
                  tunnel: [w3618 w3620] -> w3602
                  frame False {
                  }
                  frame True {
                    n2791 = Enqueue Element(queue=w3624, element="开启均衡" ("元素"), error in (no error)=w3623) -> (queue out=w3621:refnum<queue>, error out=w3620:errorcluster)  [unwired: 2 out]
                  }
                }
                n2792 = call <vilib>:"Set Busy.vi"("disable click? (T)"=TRUE) -> ()  [unwired: 3 in, 8 out]
              }
            }
          }
          event "关闭均衡": Value Change {
            n2793 = event-data() -> ("NewVal"=w3629:bool)  [unwired: 5 out]
            n2794 = case shown="真" w3629 {
              tunnel: w3628 -> [w3631 w3638]
              tunnel: w3627 -> [w3630 w3637]
              tunnel: [w3631 w3636] -> w3626
              tunnel: [w3630 w3635] -> w3625
              frame False {
              }
              frame True {
                n2795 = global read "EV05全局变量1.vi" "授权功能"() -> (w3633:bool)
                n2796 = case shown="假" w3633 {
                  tunnel: [TRUE ("发送成功") w3648] -> w3634
                  frame False {
                  }
                  frame True {
                    n2797 = local read "主从选择"() -> (w3640:enum32{"主板", "从板"})
                    n2798 = case shown="\"从板\"" w3640 {
                      tunnel: [0.0 ("FUNC") w3650] -> w3641
                      frame "主板", Default {
                      }
                      frame "从板" {
                        n2799 = local read "从板号"() -> (w3650:u8)
                      }
                    }
                    n2800 = local read "设备索引号"() -> (w3643:u16)
                    n2801 = local read "CAN卡类型"() -> (w3644:u32)
                    n2802 = local read "CAN端口"() -> (w3642:u16)
                    n2803 = call "标定授权发送.vi"("CAN卡类型"=w3644, "解锁类型"=enum16{"读取", "写", "下载"}."写", "设备索引号"=w3643, "CAN端口"=w3642, "是否连接"=TRUE, "板选择"=0, "FUNC"=w3641) -> ("发送成功"=w3648:bool)  [unwired: 8 out]
                  }
                }
                n2804 = case shown="真" w3634 {
                  tunnel: w3638 -> [w3652 w3657]
                  tunnel: w3637 -> [w3651 w3656]
                  tunnel: [w3652 w3654] -> w3636
                  tunnel: [w3651 w3653] -> w3635
                  frame False {
                  }
                  frame True {
                    n2805 = Enqueue Element(queue=w3657, element="关闭均衡" ("元素"), error in (no error)=w3656) -> (queue out=w3654:refnum<queue>, error out=w3653:errorcluster)  [unwired: 2 out]
                  }
                }
                n2806 = call <vilib>:"Set Busy.vi"("disable click? (T)"=TRUE) -> ()  [unwired: 3 in, 8 out]
              }
            }
          }
          event "强制开启均衡": Value Change {
            n2807 = event-data() -> ("NewVal"=w3662:bool)  [unwired: 5 out]
            n2808 = case shown="真" w3662 {
              tunnel: w3661 -> [w3664 w3671]
              tunnel: w3660 -> [w3663 w3670]
              tunnel: [w3664 w3669] -> w3659
              tunnel: [w3663 w3668] -> w3658
              frame False {
              }
              frame True {
                n2809 = global read "EV05全局变量1.vi" "授权功能"() -> (w3666:bool)
                n2810 = case shown="假" w3666 {
                  tunnel: [TRUE ("发送成功") w3681] -> w3667
                  frame False {
                  }
                  frame True {
                    n2811 = local read "主从选择"() -> (w3673:enum32{"主板", "从板"})
                    n2812 = case shown="\"从板\"" w3673 {
                      tunnel: [0.0 ("FUNC") w3683] -> w3674
                      frame "主板", Default {
                      }
                      frame "从板" {
                        n2813 = local read "从板号"() -> (w3683:u8)
                      }
                    }
                    n2814 = local read "设备索引号"() -> (w3676:u16)
                    n2815 = local read "CAN卡类型"() -> (w3677:u32)
                    n2816 = local read "CAN端口"() -> (w3675:u16)
                    n2817 = call "标定授权发送.vi"("CAN卡类型"=w3677, "解锁类型"=enum16{"读取", "写", "下载"}."写", "设备索引号"=w3676, "CAN端口"=w3675, "是否连接"=TRUE, "板选择"=0, "FUNC"=w3674) -> ("发送成功"=w3681:bool)  [unwired: 8 out]
                  }
                }
                n2818 = case shown="真" w3667 {
                  tunnel: w3671 -> [w3685 w3690]
                  tunnel: w3670 -> [w3684 w3689]
                  tunnel: [w3685 w3687] -> w3669
                  tunnel: [w3684 w3686] -> w3668
                  frame False {
                  }
                  frame True {
